vi "Heading.vi"(0 "X Array":dbl[](array[numeric]), 1 "Target X":dbl, 2 "Current X":dbl, 3 "Current Y":dbl, 4 "Target Y":dbl, 5 "Y Array":dbl[](array[numeric]), 7 "stop":bool) -> (6 "Current Heading":dbl, 8 "Desired Heading":dbl)   [LabVIEW 2012]
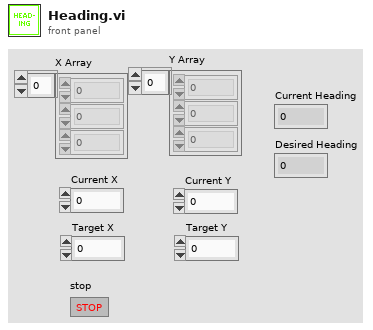
[diagram p1: front panel]
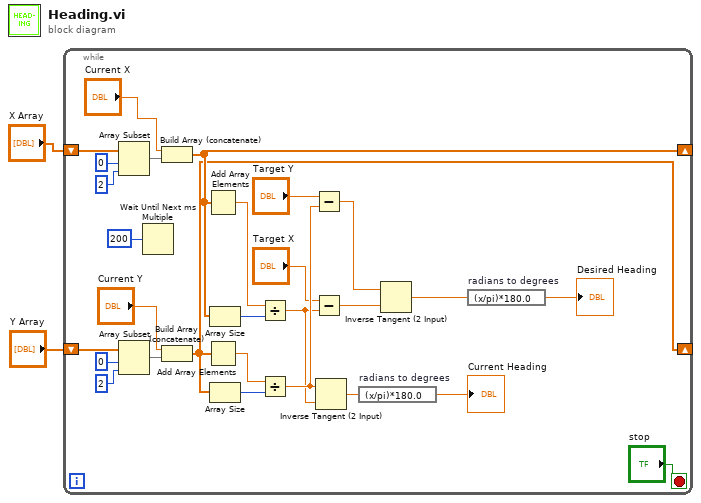
[diagram p0: block diagram]
diagram:
  n1 = while {
    shift-right: [w23] -> _
    shift-left: "X Array" -> [w30]
    shift-right: [w14] -> _
    shift-left: "Y Array" -> [w15]
    stop <- "stop" stop-if-true
    n2 = Array Subset(array=w30, index=0, length=2) -> (w27:dbl[])
    n3 = Array Subset(array=w15, index=0, length=2) -> (w19:dbl[])
    n4 = Wait Until Next ms Multiple(millisecond multiple=200) -> ()  [unwired: 1 out]
    n5 = Build Array (concatenate)("Current X", w27) -> (w23:dbl[])
    n6 = Build Array (concatenate)("Current Y", w19) -> (w14:dbl[])
    n7 = Add Array Elements(numeric array=w23) -> (sum=w24:dbl)
    n8 = Add Array Elements(numeric array=w14) -> (sum=w17:dbl)
    n9 = Array Size(array=w23) -> (size(s)=w22:i32)
    n10 = Array Size(array=w14) -> (size(s)=w16:i32)
    n11 = Divide(x=w24, y=w22) -> (x/y=w7:dbl)
    n12 = Divide(x=w17, y=w16) -> (x/y=w9:dbl)
    n13 = Subtract(x="Target Y", y=w9) -> (x-y=w11:dbl)
    n14 = Subtract(x="Target X", y=w7) -> (x-y=w6:dbl)
    n15 = Inverse Tangent (2 Input)(1:w7, 2:w9) -> (0:w13:dbl)
    n16 = expression code="(x/pi)*180.0" "radians to degrees"(w13) -> (→"Current Heading":dbl)
    n17 = Inverse Tangent (2 Input)(1:w6, 2:w11) -> (0:w5:dbl)
    n18 = expression code="(x/pi)*180.0" "radians to degrees"(w5) -> (→"Desired Heading":dbl)
  }
